vi "车牌识别.vi"(0 "请选择车牌图片":path) -> (1 "形状定位结果":string, 2 "颜色定位结果":string)   [LabVIEW 2019]
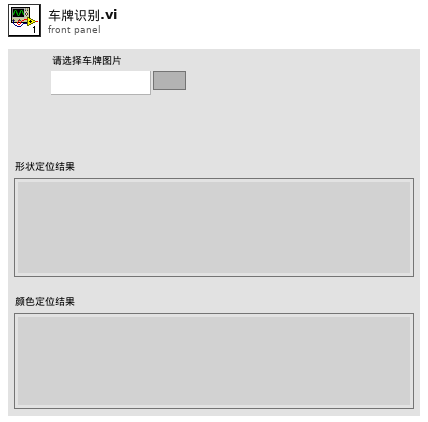
[diagram p1: front panel]
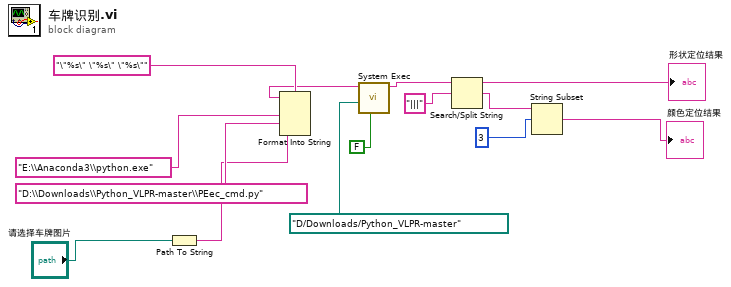
[diagram p0: block diagram]
diagram:
  n1 = Path To String(path="请选择车牌图片") -> (string=w4:string)
  n2 = Format Into String(format string="\"%s\" \"%s\" \"%s\"", "E:\\Anaconda3\\python.exe", "D:\\Downloads\\Python_VLPR-master\\PEec_cmd.py", w4) -> (resulting string=w11:string)  [unwired: 2 in, 1 out]
  n3 = call <vilib>:"System Exec.vi"("run minimized? (F)"=FALSE, "working directory"=path "D:/Downloads/Python_VLPR-master", "command line"=w11) -> ("standard output"=w9:string)  [unwired: 5 in, 3 out]
  n4 = Search/Split String(string=w9, search string/char (-)="|||") -> (substring before match=→"形状定位结果":string, match + rest of string=w6:string)  [unwired: 1 in, 1 out]
  n5 = String Subset(string=w6, offset (0)=3) -> (substring=→"颜色定位结果":string)  [unwired: 1 in]
